vi "GetOutput.vi"(8 "error in (no error)":errorcluster, 10 "test results in":T1, 11 "RunUnitTests in":refnum<class "RunUnitTests.lvclass">) -> (0 "error out":errorcluster, 1 "Output":string, 2 "Passed":bool, 3 "RunUnitTests out":refnum<class "RunUnitTests.lvclass">)   [LabVIEW 2014, in "RunUnitTests.lvclass"]
uses:
  RunUnitTests.lvclass
  <vilib>/utf/common/utf_test_result_overall.ctl
  <vilib>/utf/common/utf_test_result_testfile.ctl
  <vilib>/utf/common/utf_test_result_testcase.ctl
  <vilib>/utf/common/utf_test_result.ctl
  <vilib>/utf/common/utf_test_result_troll_new.ctl
  <vilib>/utf/common/utf_vector_result.ctl
  <vilib>/utf/common/utf_test_result_failure.ctl
  <vilib>/utf/common/utf_test_comparison_operators.ctl
  <vilib>/utf/common/utf_vi_tag.ctl
  <vilib>/utf/common/utf_test_result_input_data.ctl
  <vilib>/utf/common/utf_code_coverage.ctl
  <vilib>/utf/common/utf_error_data.ctl
  <vilib>/utf/common/utf_error_type.ctl
  <vilib>/utf/common/utf_subvi_info.ctl
  RunUnitTests.lvclass/RunUnitTests.ctl
  <vilib>/utf/NI_UnitTestFramework.lvlib
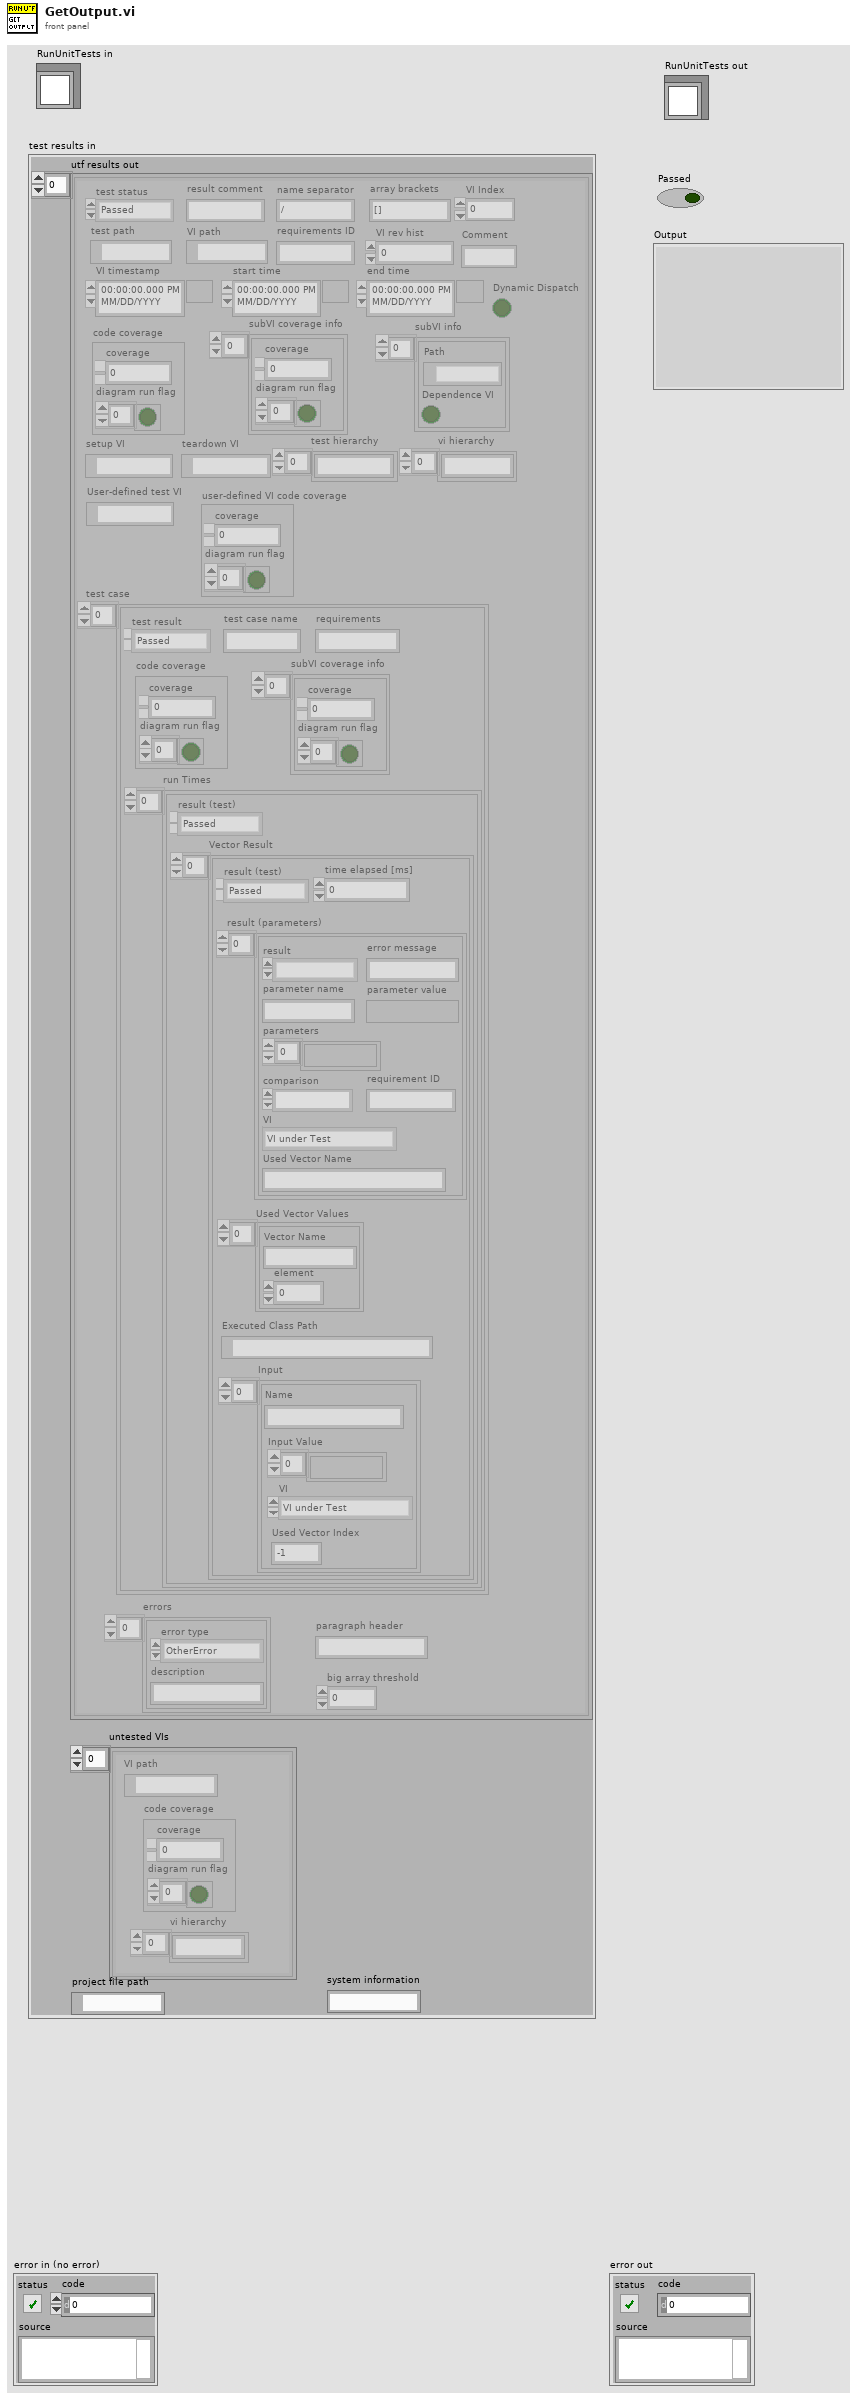
[diagram p1: front panel]
types:
  T1 = typedef "NI_UnitTestFramework.lvlib/utf_test_result_overall.ctl" = cluster{"utf results out":T2[], "untested VIs":cluster{"VI path":path, "code coverage":T11, "vi hierarchy":string[]}[], "project file path":path, "system information":string}
  T2 = typedef "NI_UnitTestFramework.lvlib/utf_test_result_testfile.ctl" = cluster{"test case":T3[], "test status":T4, "test path":path, "setup VI":path, "teardown VI":path, "code coverage":T11, "start time":timestamp, "end time":timestamp, "test hierarchy":string[], "VI path":path, "VI timestamp":timestamp, "VI rev hist":i32, "requirements ID":string, "array brackets":string, "name separator":string, "errors":T12[], "paragraph header":string, "result comment":string, "vi hierarchy":string[], "subVI coverage info":T11[], "subVI info":T14[], "big array threshold":u32, "VI Index":i32, "Comment":string, "Dynamic Dispatch":bool, "User-defined test VI":path, "user-defined VI code coverage":T11}
  T3 = typedef "NI_UnitTestFramework.lvlib/utf_test_result_testcase.ctl" = cluster{"test result":T4, "run Times":T5[], "test case name":string, "requirements":string, "code coverage":T11, "subVI coverage info":T11[]}
  T4 = typedef "NI_UnitTestFramework.lvlib/utf_test_result.ctl" = enum16{"Passed", "Failed", "Error", "Skipped", "Not Processed"}
  T5 = typedef "NI_UnitTestFramework.lvlib/utf_test_result_troll_new.ctl" = cluster{"result (test)":T4, "Vector Result":T6[]}
  T6 = typedef "NI_UnitTestFramework.lvlib/utf_vector_result.ctl" = cluster{"time elapsed [ms]":u32, "result (test)":T4, "result (parameters)":T7[], "Used Vector Values":cluster{"Vector Name":string, "element":i32}[], "Executed Class Path":path, "Input":T10[]}
  T7 = typedef "NI_UnitTestFramework.lvlib/utf_test_result_failure.ctl" = cluster{"result":T4, "error message":string, "parameter name":string, "parameter value":variant, "parameters":variant[], "comparison":T8, "requirement ID":string, "VI":T9, "Used Vector Name":string}
  T8 = typedef "NI_UnitTestFramework.lvlib/utf_test_comparison_operators.ctl" = enum16{"=", "!=", ">", ">=", "<", "<=", "range", "symmetric tolerance", "asymmetric tolerance", "string contains", "string not contain", "array size", "string length", "array range", "by element", "array range (limit array)", "user-defined", "array contains", "array not contain", "vector length", "= (elm)", "!= (elm)", "= (case insensitive)", "!= (case insensitive)"}
  T9 = typedef "NI_UnitTestFramework.lvlib/utf_vi_tag.ctl" = enum16{"Setup VI", "VI under Test", "Teardown VI"}
  T10 = typedef "NI_UnitTestFramework.lvlib/utf_test_result_input_data.ctl" = cluster{"Name":string, "Input Value":variant[], "VI":T9, "Used Vector Index":i32}
  T11 = typedef "NI_UnitTestFramework.lvlib/utf_code_coverage.ctl" = cluster{"coverage":dbl, "diagram run flag":bool[]}
  T12 = typedef "NI_UnitTestFramework.lvlib/utf_error_data.ctl" = cluster{"error type":T13, "description":string}
  T13 = typedef "NI_UnitTestFramework.lvlib/utf_error_type.ctl" = enum16{"TestFileError", "VIError", "SetupVIError", "TearDownVIError", "OtherError"}
  T14 = typedef "NI_UnitTestFramework.lvlib/utf_subvi_info.ctl" = cluster{"Path":path, "Dependence VI":bool}
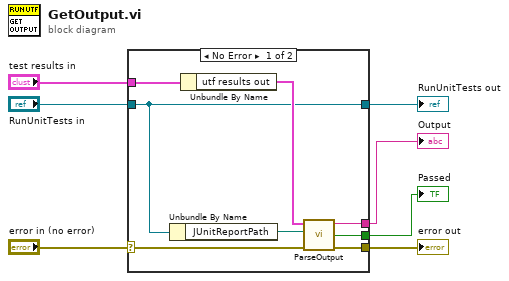
[diagram p0: block diagram]
diagram:
  n1 = case shown="No Error" "error in (no error)" {
    selector: "error in (no error)" -> [w13 w17]
    tunnel: [w9 w17] -> w7
    tunnel: "test results in" -> [w14 _]
    tunnel: "RunUnitTests in" -> [w12 w16]
    tunnel: [w12 w16] -> w3
    tunnel: [w8 _] -> w2
    tunnel: [w11 _] -> w1
    frame No Error {
      n2 = Unbundle By Name(w12) -> ("JUnitReportPath"=w10:path)
      n3 = Unbundle By Name(w14) -> ("utf results out"=w15:T2[])
      n4 = call "ParseOutput.vi"("error in (no error)"=w13, "JUnit report path"=w10, "utf results in"=w15) -> ("error out"=w9:errorcluster, "Passed?"=w11:bool, "Output"=w8:string)  [unwired: 6 in]
    }
    frame Error {
    }
  }
  "Output" <- w2
  "error out" <- w7
  "Passed" <- w1
  "RunUnitTests out" <- w3
